vi "Transpose Matrix.vi"   [LabVIEW 2010, in "NI_AALPro.lvlib"]
doc: "Transposes <B>Input Matrix</B>. If <B>Input Matrix</B> is a complex matrix, the VI performs conjugate transposition. Wire data to the <B>Input Matrix</B> input to determine the polymorphic instance to use or manually select the instance."
uses:
  NI_AALPro.lvlib
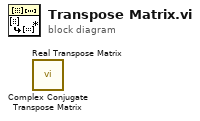
[diagram p0: block diagram]
diagram:
  n1 = call "Complex Conjugate Transpose Matrix.vi"() -> ()  [unwired: 10 in, 2 out]
  n2 = call "Real Transpose Matrix.vi"() -> ()  [unwired: 10 in, 2 out]
